vi "Write KPRO Data cells to excel.vi"(0 "NI_report in":refnum<class "NI_report.lvclass">, 1 "milliseconds to wait":u32=100, 2 "all rows":string[][](array[string]), 3 "Row Offset In":i32=2, 5 "error in (no error)":errorcluster, 6 "Worksheet Names":string[](array[string])) -> (14 "NI_report out":refnum<class "NI_report.lvclass">, 16 "Row Offset Out":i32, 19 "error out":errorcluster)   [LabVIEW 2016]
uses:
  <vilib>/Utility/NIReport.llb/NI_report.lvclass
panel:
  out "number of rows":i32
  out "size(s)":i32[](array[numeric])
  in  "Current Sample Sheet":string="Processed Ik"
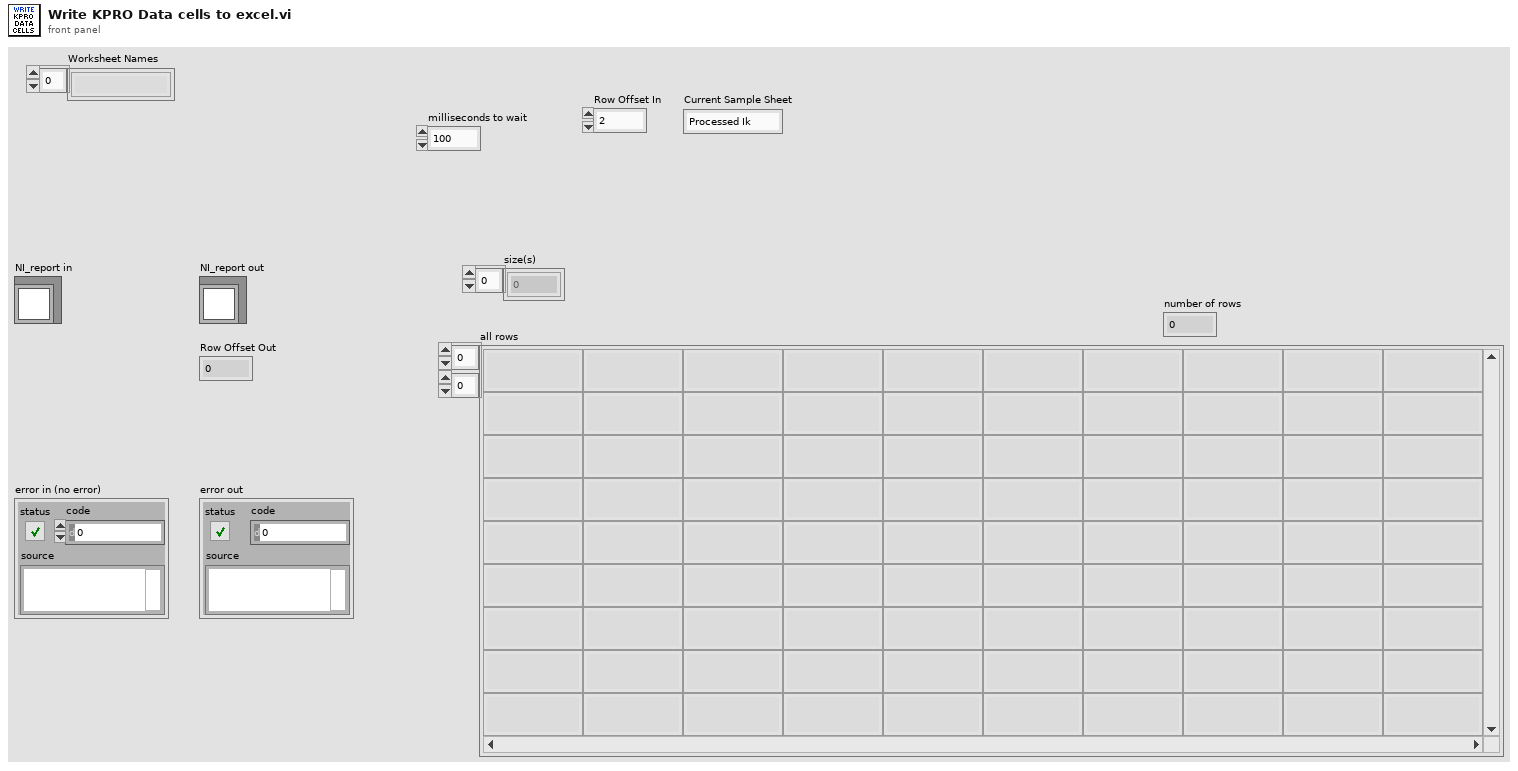
[diagram p1: front panel]
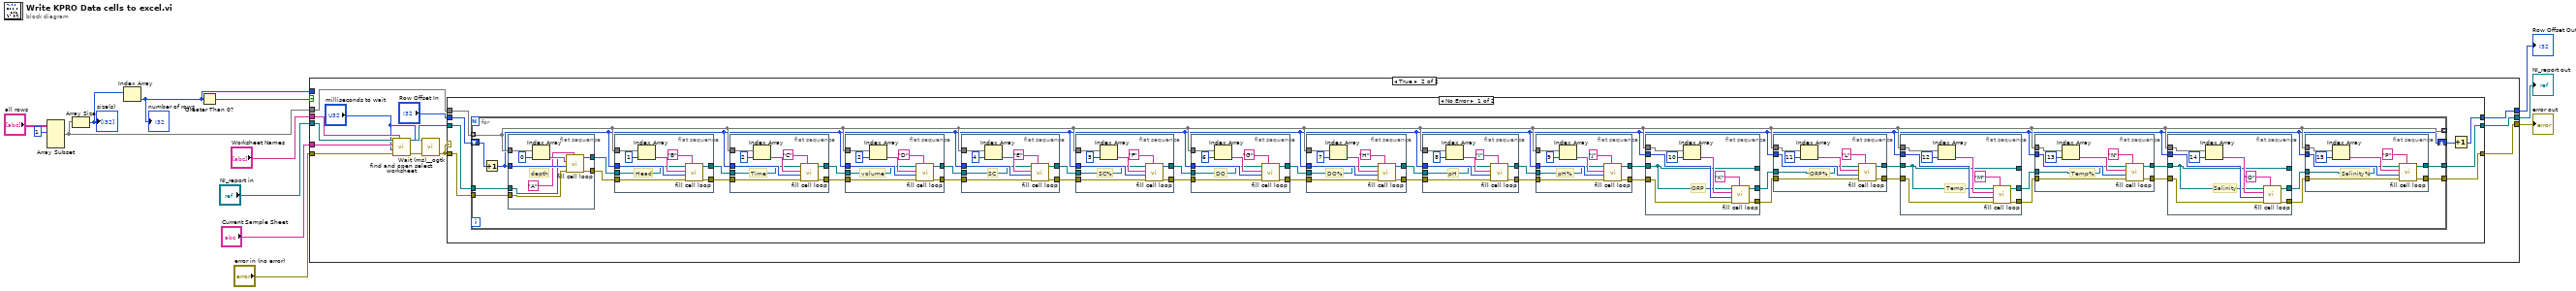
[diagram p0: block diagram]
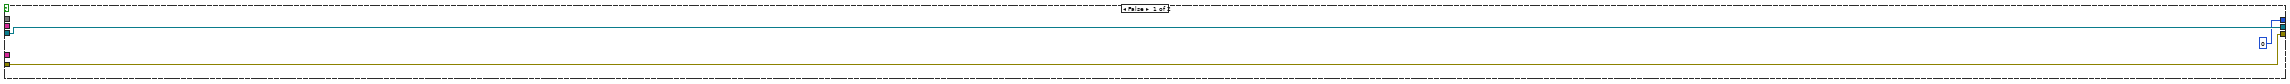
[diagram p2: hidden frame]
diagram:
  n1 = Array Subset(array="all rows", index (row)=1 ("index")) -> (w4:string[][])  [unwired: 3 in]
  n2 = Array Size(array=w4) -> (size(s)=w3:i32[])
  "size(s)" <- w3
  n3 = Index Array(array=w3) -> (element=w2:i32)  [unwired: 1 in]
  "number of rows" <- w2
  n4 = Greater Than 0?(x=w2) -> (x > 0?=w8:bool)
  n5 = case shown="True" w8 {
    tunnel: [w15 w29] -> w13
    tunnel: [w16 w28] -> w12
    tunnel: [0 ("Row Offset In") w18] -> w11
    tunnel: "NI_report in" -> [w16 w25]
    tunnel: "error in (no error)" -> [w15 w21]
    tunnel: "Worksheet Names" -> [_ w24]
    tunnel: w4 -> [_ w26]
    tunnel: w2 -> [_ _]
    tunnel: "Current Sample Sheet" -> [_ w20]
    frame False {
    }
    frame True {
      n6 = call "find and open select worksheet.vi"("Worksheet Names"=w24, "error in (no error)"=w21, "milliseconds to wait"="milliseconds to wait", "Worksheet Name in"=w20, "NI_report in"=w25) -> ("error out"=w22:errorcluster, "NI_report out"=w23:refnum<class "NI_report.lvclass">)  [unwired: 4 in, 1 out]
      n7 = call <userlib>:"Wait (ms)__ogtk.vi"("error in (no error)"=w22, "milliseconds to wait"="milliseconds to wait") -> ("error out"=w17:errorcluster)  [unwired: 8 in, 1 out]
      n8 = case shown="No Error" w17 {
        tunnel: [w37 w221] -> w29
        tunnel: [w36 w219] -> w28
        tunnel: "Row Offset In" -> [w34 w220]
        tunnel: w26 -> [w33 _]
        tunnel: w23 -> [w32 w219]
        tunnel: w17 -> [w31 w221]
        tunnel: [w30 w220] -> w18
        frame No Error {
          n9 = for {
            tunnel: w33 -> [w41] mode=indexing
            shift-right: [w40] -> w35
            shift-left: w34 -> [w74]
            tunnel: w32 -> [w71]
            tunnel: w31 -> [w73]
            tunnel: [w39] -> w37
            tunnel: [w38] -> w36
            tunnel: [w41] -> _ mode=indexing
            n10 = Increment(x=w74) -> (x+1=w40:i32)
            n11 = flat-sequence {
              tunnel: w41 -> [w217]
              tunnel: w73 -> [w216]
              tunnel: [w215] -> w72
              tunnel: w40 -> [w214]
              tunnel: w71 -> [w212]
              tunnel: [w211] -> w70
              frame #0 {
                # "depth"
                n12 = Index Array(array=w217, index=0) -> (element=w213:string)
                n13 = call "fill cell loop.vi"("Column Letter"="A" ("Depth Column Letter"), "error in (no error)"=w216, "Row"=w214, "String"=w213, "NI_report in"=w212) -> ("error out"=w215:errorcluster, "NI_report out"=w211:refnum<class "NI_report.lvclass">)  [unwired: 5 in]
              }
            }
            n14 = flat-sequence {
              tunnel: [w209] -> w68
              tunnel: [w208] -> w69
              tunnel: w41 -> [w204]
              tunnel: w72 -> [w203]
              tunnel: w40 -> [w202]
              tunnel: w70 -> [w201]
              frame #0 {
                # "Head"
                n15 = Index Array(array=w204, index=1) -> (element=w205:string)
                n16 = call "fill cell loop.vi"("Column Letter"="B" ("Head Column Letter"), "error in (no error)"=w203, "Row"=w202, "String"=w205, "NI_report in"=w201) -> ("error out"=w209:errorcluster, "NI_report out"=w208:refnum<class "NI_report.lvclass">)  [unwired: 5 in]
              }
            }
            n17 = flat-sequence {
              tunnel: [w200] -> w66
              tunnel: [w199] -> w67
              tunnel: w41 -> [w195]
              tunnel: w68 -> [w194]
              tunnel: w40 -> [w193]
              tunnel: w69 -> [w192]
              frame #0 {
                # "Time"
                n18 = Index Array(array=w195, index=2) -> (element=w196:string)
                n19 = call "fill cell loop.vi"("Column Letter"="C" ("Head Column Letter"), "error in (no error)"=w194, "Row"=w193, "String"=w196, "NI_report in"=w192) -> ("error out"=w200:errorcluster, "NI_report out"=w199:refnum<class "NI_report.lvclass">)  [unwired: 5 in]
              }
            }
            n20 = flat-sequence {
              tunnel: [w191] -> w64
              tunnel: [w190] -> w65
              tunnel: w41 -> [w186]
              tunnel: w66 -> [w185]
              tunnel: w40 -> [w184]
              tunnel: w67 -> [w183]
              frame #0 {
                # "volume"
                n21 = Index Array(array=w186, index=2) -> (element=w187:string)
                n22 = call "fill cell loop.vi"("Column Letter"="D" ("Head Column Letter"), "error in (no error)"=w185, "Row"=w184, "String"=w187, "NI_report in"=w183) -> ("error out"=w191:errorcluster, "NI_report out"=w190:refnum<class "NI_report.lvclass">)  [unwired: 5 in]
              }
            }
            n23 = flat-sequence {
              tunnel: [w182] -> w62
              tunnel: [w181] -> w63
              tunnel: w41 -> [w177]
              tunnel: w64 -> [w176]
              tunnel: w40 -> [w175]
              tunnel: w65 -> [w174]
              frame #0 {
                # "SC"
                n24 = Index Array(array=w177, index=4) -> (element=w178:string)
                n25 = call "fill cell loop.vi"("Column Letter"="E" ("Head Column Letter"), "error in (no error)"=w176, "Row"=w175, "String"=w178, "NI_report in"=w174) -> ("error out"=w182:errorcluster, "NI_report out"=w181:refnum<class "NI_report.lvclass">)  [unwired: 5 in]
              }
            }
            n26 = flat-sequence {
              tunnel: [w173] -> w58
              tunnel: [w172] -> w59
              tunnel: w41 -> [w168]
              tunnel: w62 -> [w167]
              tunnel: w40 -> [w166]
              tunnel: w63 -> [w165]
              frame #0 {
                # "SC%"
                n27 = Index Array(array=w168, index=5) -> (element=w169:string)
                n28 = call "fill cell loop.vi"("Column Letter"="F" ("Head Column Letter"), "error in (no error)"=w167, "Row"=w166, "String"=w169, "NI_report in"=w165) -> ("error out"=w173:errorcluster, "NI_report out"=w172:refnum<class "NI_report.lvclass">)  [unwired: 5 in]
              }
            }
            n29 = flat-sequence {
              tunnel: [w164] -> w61
              tunnel: [w163] -> w60
              tunnel: w41 -> [w159]
              tunnel: w58 -> [w158]
              tunnel: w40 -> [w157]
              tunnel: w59 -> [w156]
              frame #0 {
                # "DO"
                n30 = Index Array(array=w159, index=6) -> (element=w160:string)
                n31 = call "fill cell loop.vi"("Column Letter"="G" ("Head Column Letter"), "error in (no error)"=w158, "Row"=w157, "String"=w160, "NI_report in"=w156) -> ("error out"=w164:errorcluster, "NI_report out"=w163:refnum<class "NI_report.lvclass">)  [unwired: 5 in]
              }
            }
            n32 = flat-sequence {
              tunnel: [w155] -> w54
              tunnel: [w154] -> w55
              tunnel: w41 -> [w150]
              tunnel: w61 -> [w149]
              tunnel: w40 -> [w148]
              tunnel: w60 -> [w147]
              frame #0 {
                # "DO%"
                n33 = Index Array(array=w150, index=7) -> (element=w151:string)
                n34 = call "fill cell loop.vi"("Column Letter"="H" ("Head Column Letter"), "error in (no error)"=w149, "Row"=w148, "String"=w151, "NI_report in"=w147) -> ("error out"=w155:errorcluster, "NI_report out"=w154:refnum<class "NI_report.lvclass">)  [unwired: 5 in]
              }
            }
            n35 = flat-sequence {
              tunnel: [w146] -> w56
              tunnel: [w145] -> w57
              tunnel: w41 -> [w141]
              tunnel: w54 -> [w140]
              tunnel: w40 -> [w139]
              tunnel: w55 -> [w138]
              frame #0 {
                # "pH"
                n36 = Index Array(array=w141, index=8) -> (element=w142:string)
                n37 = call "fill cell loop.vi"("Column Letter"="I" ("Head Column Letter"), "error in (no error)"=w140, "Row"=w139, "String"=w142, "NI_report in"=w138) -> ("error out"=w146:errorcluster, "NI_report out"=w145:refnum<class "NI_report.lvclass">)  [unwired: 5 in]
              }
            }
            n38 = flat-sequence {
              tunnel: [w137] -> w51
              tunnel: [w136] -> w50
              tunnel: w41 -> [w132]
              tunnel: w56 -> [w131]
              tunnel: w40 -> [w130]
              tunnel: w57 -> [w129]
              frame #0 {
                # "pH%"
                n39 = Index Array(array=w132, index=9) -> (element=w133:string)
                n40 = call "fill cell loop.vi"("Column Letter"="J" ("Head Column Letter"), "error in (no error)"=w131, "Row"=w130, "String"=w133, "NI_report in"=w129) -> ("error out"=w137:errorcluster, "NI_report out"=w136:refnum<class "NI_report.lvclass">)  [unwired: 5 in]
              }
            }
            n41 = flat-sequence {
              tunnel: [w128] -> w53
              tunnel: [w127] -> w52
              tunnel: w41 -> [w123]
              tunnel: w51 -> [w122]
              tunnel: w40 -> [w121]
              tunnel: [w120] -> _
              tunnel: w50 -> [w120]
              frame #0 {
                # "ORP"
                n42 = Index Array(array=w123, index=10) -> (element=w124:string)
                n43 = call "fill cell loop.vi"("Column Letter"="K" ("Head Column Letter"), "error in (no error)"=w122, "Row"=w121, "String"=w124, "NI_report in"=w120) -> ("error out"=w128:errorcluster, "NI_report out"=w127:refnum<class "NI_report.lvclass">)  [unwired: 5 in]
              }
            }
            n44 = flat-sequence {
              tunnel: [w119] -> w47
              tunnel: [w118] -> w46
              tunnel: w41 -> [w114]
              tunnel: w53 -> [w113]
              tunnel: w40 -> [w112]
              tunnel: w52 -> [w111]
              frame #0 {
                # "ORP%"
                n45 = Index Array(array=w114, index=11) -> (element=w115:string)
                n46 = call "fill cell loop.vi"("Column Letter"="L" ("Head Column Letter"), "error in (no error)"=w113, "Row"=w112, "String"=w115, "NI_report in"=w111) -> ("error out"=w119:errorcluster, "NI_report out"=w118:refnum<class "NI_report.lvclass">)  [unwired: 5 in]
              }
            }
            n47 = flat-sequence {
              tunnel: [w92] -> w43
              tunnel: [w91] -> w42
              tunnel: w41 -> [w87]
              tunnel: w47 -> [w86]
              tunnel: w40 -> [w85]
              tunnel: w46 -> [w84]
              tunnel: [w84] -> _
              frame #0 {
                # "Temp"
                n48 = Index Array(array=w87, index=12) -> (element=w88:string)
                n49 = call "fill cell loop.vi"("Column Letter"="M" ("Head Column Letter"), "error in (no error)"=w86, "Row"=w85, "String"=w88, "NI_report in"=w84) -> ("error out"=w92:errorcluster, "NI_report out"=w91:refnum<class "NI_report.lvclass">)  [unwired: 5 in]
              }
            }
            n50 = flat-sequence {
              tunnel: [w83] -> w44
              tunnel: [w82] -> w45
              tunnel: w41 -> [w78]
              tunnel: w40 -> [w77]
              tunnel: w43 -> [w76]
              tunnel: w42 -> [w75]
              frame #0 {
                # "Temp%"
                n51 = Index Array(array=w78, index=13) -> (element=w79:string)
                n52 = call "fill cell loop.vi"("Column Letter"="N" ("Head Column Letter"), "error in (no error)"=w76, "Row"=w77, "String"=w79, "NI_report in"=w75) -> ("error out"=w83:errorcluster, "NI_report out"=w82:refnum<class "NI_report.lvclass">)  [unwired: 5 in]
              }
            }
            n53 = flat-sequence {
              tunnel: [w110] -> w48
              tunnel: [w109] -> w49
              tunnel: w41 -> [w105]
              tunnel: w44 -> [w104]
              tunnel: w40 -> [w103]
              tunnel: w45 -> [w102]
              tunnel: [w102] -> _
              frame #0 {
                # "Salinity"
                n54 = Index Array(array=w105, index=14) -> (element=w106:string)
                n55 = call "fill cell loop.vi"("Column Letter"="O" ("Head Column Letter"), "error in (no error)"=w104, "Row"=w103, "String"=w106, "NI_report in"=w102) -> ("error out"=w110:errorcluster, "NI_report out"=w109:refnum<class "NI_report.lvclass">)  [unwired: 5 in]
              }
            }
            n56 = flat-sequence {
              tunnel: [w101] -> w39
              tunnel: [w100] -> w38
              tunnel: w41 -> [w96]
              tunnel: w48 -> [w95]
              tunnel: w40 -> [w94]
              tunnel: w49 -> [w93]
              frame #0 {
                # "Salinity%"
                n57 = Index Array(array=w96, index=15) -> (element=w97:string)
                n58 = call "fill cell loop.vi"("Column Letter"="P" ("Head Column Letter"), "error in (no error)"=w95, "Row"=w94, "String"=w97, "NI_report in"=w93) -> ("error out"=w101:errorcluster, "NI_report out"=w100:refnum<class "NI_report.lvclass">)  [unwired: 5 in]
              }
            }
          }
          n59 = Increment(x=w35) -> (x+1=w30:i32)
        }
        frame Error {
        }
      }
    }
  }
  "error out" <- w13
  "NI_report out" <- w12
  "Row Offset Out" <- w11
